vi "Cell Enable All.vi"(7 "Box ID":u8, 8 "error in (no error)":errorcluster, 10 "Enable":bool, 11 "ENET in":refnum<class "ENET_BS120x.lvclass">) -> (0 "error out":errorcluster, 3 "ENET out":refnum<class "ENET_BS120x.lvclass">)   [LabVIEW 2021, in "BS120x Driver.lvlib" / "ENET_BS120x.lvclass"]
uses:
  ENET_BS120x.lvclass
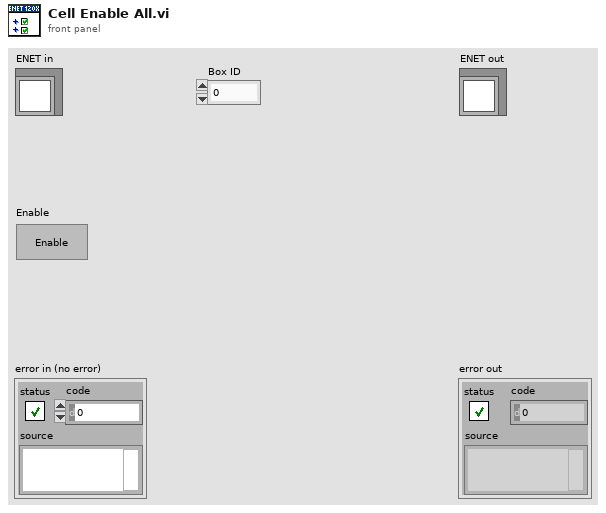
[diagram p1: front panel]
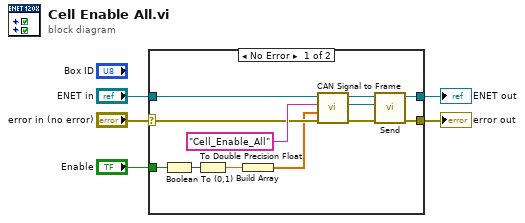
[diagram p0: block diagram]
diagram:
  n1 = case shown="No Error" "error in (no error)" {
    selector: "error in (no error)" -> [w12 w18]
    tunnel: [w13 w18] -> w5
    tunnel: "Enable" -> [w9 _]
    tunnel: "ENET in" -> [w7 w19]
    tunnel: [w6 w19] -> w1
    frame No Error {
      n2 = Boolean To (0,1)(Boolean=w9) -> (0, 1=w11:i16)
      n3 = To Double Precision Float(number=w11) -> (double precision float=w10:dbl)
      n4 = Build Array(w10) -> (w8:dbl[])
      n5 = call "CAN Signal to Frame.vi"("error in (no error)"=w12, "Data Array"=w8, "Frame"="Cell_Enable_All", "ENET in"=w7) -> ("error out"=w14:errorcluster, "Data"=w15:refnum<class "Data.lvclass">, "ENET out"=w16:refnum<class "ENET_BS120x.lvclass">)  [unwired: 5 in]
      n6 = call "Send.vi"("error in (no error)"=w14, "Data"=w15, "ENET in"=w16) -> ("error out"=w13:errorcluster, "ENET out"=w6:refnum<class "ENET_BS120x.lvclass">)  [unwired: 7 in]
    }
    frame Error {
    }
  }
  "error out" <- w5
  "ENET out" <- w1
